vi "Manual.vi"(8 "error in (no error)":errorcluster, 10 "shutdown":refnum<user-event>, 11 "Modules":T2) -> (0 "Error 2":errorcluster)   [LabVIEW 2025]
uses:
  <vilib>/Handler Framework/CmdQueue/Enqueue Single.vi
  <vilib>/Handler Framework/Handler Framework.lvlib
  Libraries/USB IO/Classes/Hardware Selection.ctl
  Controls/Test list.ctl
panel:
  in  "Cluster 2":T1
  out "Module Names":string[](array[string])
  out "Error":errorcluster
  # "Manual"
  # "Test"
  # "Wear-in"
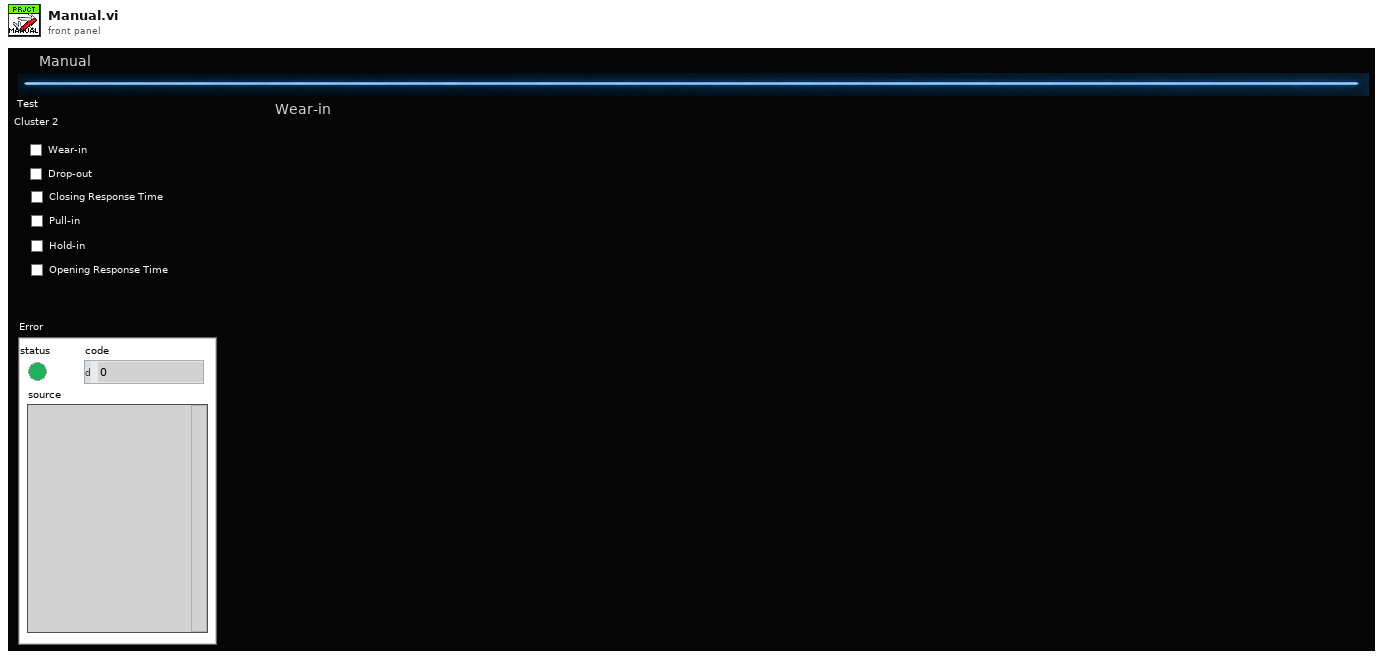
[diagram p1: front panel]
types:
  T1 = typedef "Test list.ctl" = cluster{"Wear-in":bool, "Drop-out":bool, "Closing Response Time":bool, "Pull-in":bool, "Hold-in":bool, "Opening Response Time":bool}
  T2 = cluster{"Module IDs":i32[], "Module Names":string[]}
  T3 = typedef "Hardware Selection.ctl" = enum16{"Simulation", "USB-6000", "USB-6001", "Arduino Uno"}
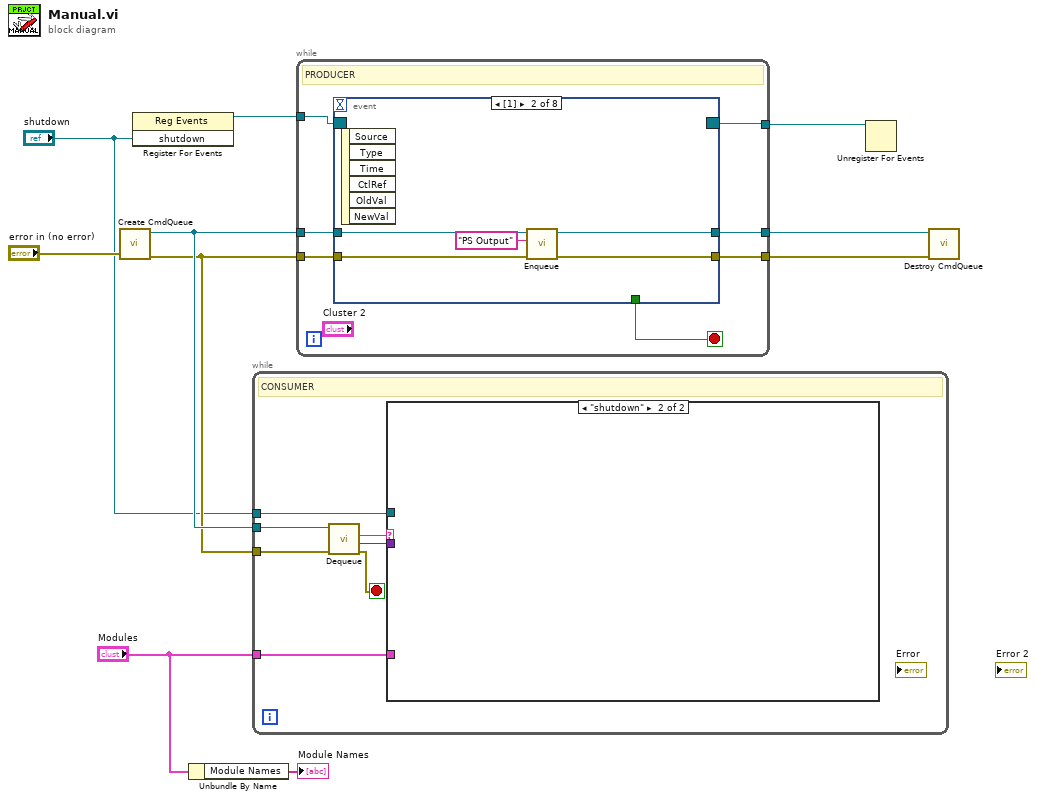
[diagram p0: block diagram]
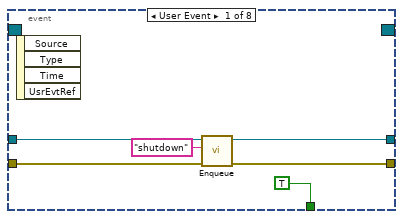
[diagram p3: hidden frame]
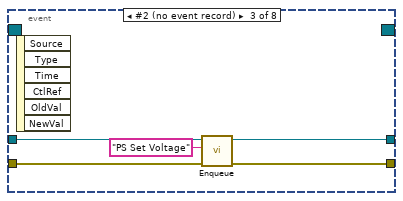
[diagram p4: hidden frame]
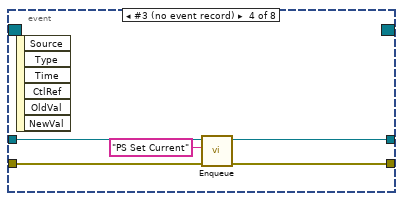
[diagram p5: hidden frame]
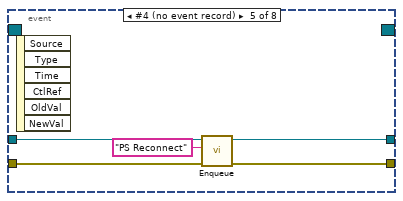
[diagram p6: hidden frame]
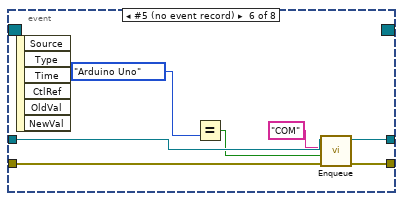
[diagram p7: hidden frame]
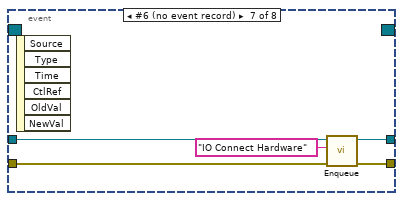
[diagram p8: hidden frame]
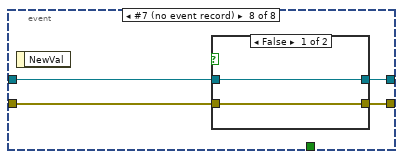
[diagram p9: hidden frame]
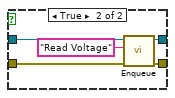
[diagram p10: hidden frame]
diagram:
  n1 = call <vilib>:"Create CmdQueue.vi"("error in (no error)"="error in (no error)") -> ("error out"=w7:errorcluster, "CmdQueue out"=w8:refnum<queue>)  [unwired: 9 in]
  n2 = register-events("shutdown") -> (reference out=w6:refnum<event-registration>)  [unwired: 2 in, 1 out]
  n3 = Unbundle By Name("Modules") -> ("Module Names"=→"Module Names":string[])
  n4 = while {
    tunnel: w8 -> [w17]
    tunnel: w7 -> [w13]
    tunnel: "shutdown" -> [w12]
    tunnel: "Modules" -> [w11]
    stop <- w14 stop-if-true
    # "CONSUMER"
    n5 = call <vilib>:"Dequeue.vi"("error in (no error)"=w13, "CmdQueue in"=w17) -> ("error out"=w14:errorcluster, "value"=w15:variant, "cmd"=w16:string)  [unwired: 5 in, 2 out]
    n6 = case shown="\"shutdown\"" w16 {
      tunnel: w15 -> [_ _]
      tunnel: w12 -> [_ _]
      tunnel: w11 -> [_ _]
      frame "init" {
      }
      frame "shutdown" {
      }
    }
  }
  n7 = while {
    tunnel: w8 -> [w24]
    tunnel: [w23] -> w10
    tunnel: w7 -> [w22]
    tunnel: [w21] -> w9
    tunnel: w6 -> [w19]
    tunnel: [w18] -> w5
    stop <- w20 stop-if-true
    # "PRODUCER"
    n8 = event shown="[1]" {
      selector: w19 -> [_ _ _ _ _ _ _ _]
      dyn-events: [_ _ _ _ _ _ _ _] -> w18
      timeout: _ -> [_ _ _ _ _ _ _ _]
      tunnel: w24 -> [w30 w35 w40 w45 w50 w54 w60 w64]
      tunnel: [w29 w34 w39 w44 w49 w55 w61 w65] -> w23
      tunnel: w22 -> [w28 w33 w38 w43 w48 w53 w59 w63]
      tunnel: [w27 w32 w37 w42 w47 w56 w62 w66] -> w21
      tunnel: [TRUE ("Discard?") _ _ _ _ _ _ _] -> w20
      event User Event {
        n9 = event-data() -> ()  [unwired: 1 in, 4 out]
        n10 = call-poly <vilib>:"Enqueue.vi"("error in (no error)"=w28, "Command"="shutdown", "CmdQueue in"=w30) -> ("error out"=w27:errorcluster, "CmdQueue out"=w29:refnum<queue>)  [unwired: 7 in]
      }
      event #1 (no event record) {
        n11 = event-data() -> ()  [unwired: 1 in, 6 out]
        n12 = call-poly <vilib>:"Enqueue.vi"("error in (no error)"=w33, "Command"="PS Output", "CmdQueue in"=w35) -> ("error out"=w32:errorcluster, "CmdQueue out"=w34:refnum<queue>)  [unwired: 7 in]
      }
      event #2 (no event record) {
        n13 = event-data() -> ()  [unwired: 1 in, 6 out]
        n14 = call-poly <vilib>:"Enqueue.vi"("error in (no error)"=w38, "Command"="PS Set Voltage", "CmdQueue in"=w40) -> ("error out"=w37:errorcluster, "CmdQueue out"=w39:refnum<queue>)  [unwired: 7 in]
      }
      event #3 (no event record) {
        n15 = event-data() -> ()  [unwired: 1 in, 6 out]
        n16 = call-poly <vilib>:"Enqueue.vi"("error in (no error)"=w43, "Command"="PS Set Current", "CmdQueue in"=w45) -> ("error out"=w42:errorcluster, "CmdQueue out"=w44:refnum<queue>)  [unwired: 7 in]
      }
      event #4 (no event record) {
        n17 = event-data() -> ()  [unwired: 1 in, 6 out]
        n18 = call-poly <vilib>:"Enqueue.vi"("error in (no error)"=w48, "Command"="PS Reconnect", "CmdQueue in"=w50) -> ("error out"=w47:errorcluster, "CmdQueue out"=w49:refnum<queue>)  [unwired: 7 in]
      }
      event #5 (no event record) {
        n19 = event-data() -> ()  [unwired: 1 in, 6 out]
        n20 = Equal?(y=Hardware_Selection."Arduino Uno" ("NewVal")) -> (x = y?=w51:bool)  [unwired: 1 in]
        n21 = call-poly <vilib>:"Enqueue.vi"("error in (no error)"=w53, "Value"=w51, "Command"="COM", "CmdQueue in"=w54) -> ("error out"=w56:errorcluster, "CmdQueue out"=w55:refnum<queue>)  [unwired: 6 in]
      }
      event #6 (no event record) {
        n22 = event-data() -> ()  [unwired: 1 in, 6 out]
        n23 = call-poly <vilib>:"Enqueue.vi"("error in (no error)"=w59, "Command"="IO Connect Hardware", "CmdQueue in"=w60) -> ("error out"=w62:errorcluster, "CmdQueue out"=w61:refnum<queue>)  [unwired: 7 in]
      }
      event #7 (no event record) {
        n24 = event-data() -> ()  [unwired: 1 in, 1 out]
        n25 = case shown="False" {
          selector: _ -> [_ _]
          tunnel: [w67 w73] -> w66
          tunnel: [w68 w72] -> w65
          tunnel: w64 -> [w68 w71]
          tunnel: w63 -> [w67 w70]
          frame False {
          }
          frame True {
            n26 = call-poly <vilib>:"Enqueue.vi"("error in (no error)"=w70, "Command"="Read Voltage", "CmdQueue in"=w71) -> ("error out"=w73:errorcluster, "CmdQueue out"=w72:refnum<queue>)  [unwired: 7 in]
          }
        }
      }
    }
  }
  n27 = Unregister For Events(event registration refnum=w5) -> ()  [unwired: 1 in, 1 out]
  n28 = call <vilib>:"Destroy CmdQueue.vi"("error in (no error)"=w9, "CmdQueue in"=w10) -> ()  [unwired: 9 in, 1 out]
